vi "deleteTempFiles.vi"(6 "error in":errorcluster, 9 "path":path) -> (0 "error out":errorcluster)   [LabVIEW 2012]
panel:
  out "deleting":path
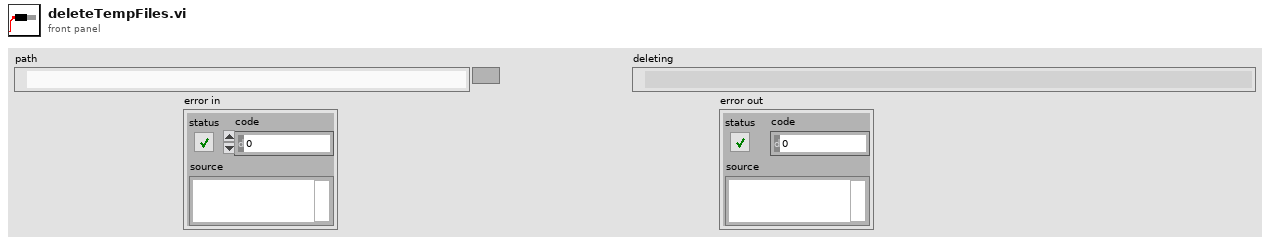
[diagram p1: front panel]
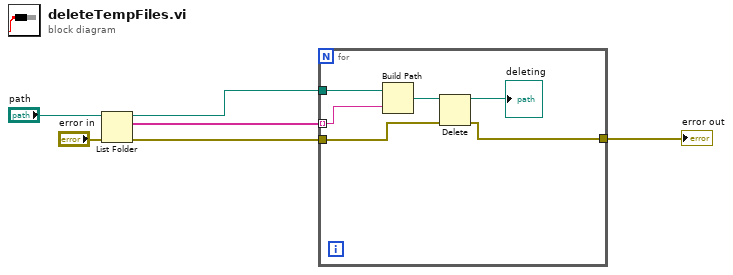
[diagram p0: block diagram]
diagram:
  n1 = List Folder(path="path", error in="error in") -> (path out=w4:path, filenames=w5:string[], error out=w2:errorcluster)  [unwired: 2 in, 1 out]
  n2 = for {
    tunnel: w5 -> [w11] mode=indexing
    tunnel: w4 -> [w12]
    tunnel: w2 -> [w8]
    tunnel: [w7] -> w1
    n3 = Build Path(base path=w12, name or relative path=w11) -> (appended path=w10:path)
    n4 = Delete(path (use dialog)=w10, error in=w8) -> (deleted path=→"deleting":path, error out=w7:errorcluster)  [unwired: 3 in, 1 out]
  }
  "error out" <- w1
